vi "Measure Triggered Suply IV.vi"(0 "Supply Line Handle in":refnum<k15>, 1 "Channel Name":string, 11 "error in (no error)":errorcluster) -> (4 "Supply Line Handle out":refnum<k15>, 6 "Supply Line Measurements Results":T1, 15 "error out":errorcluster)   [LabVIEW 2016, in "SMU.lvlib"]
uses:
  SMU.lvlib
  <instrlib>/niDCPower/nidcpower.llb/niDCPower Send Software Edge Trigger - Signal.ctl
  Typedefs/IV Results.ctl
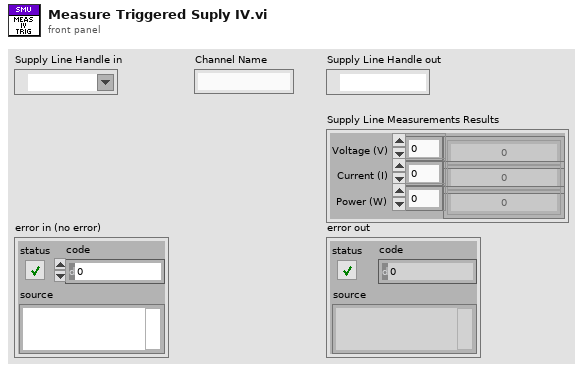
[diagram p1: front panel]
types:
  T1 = typedef "SMU.lvlib/IV Results.ctl" = cluster{"Voltage (V)":dbl[], "Current (I)":dbl[], "Power (W)":dbl[]}
  T2 = typedef "niDCPower Send Software Edge Trigger - Signal.ctl" = i32
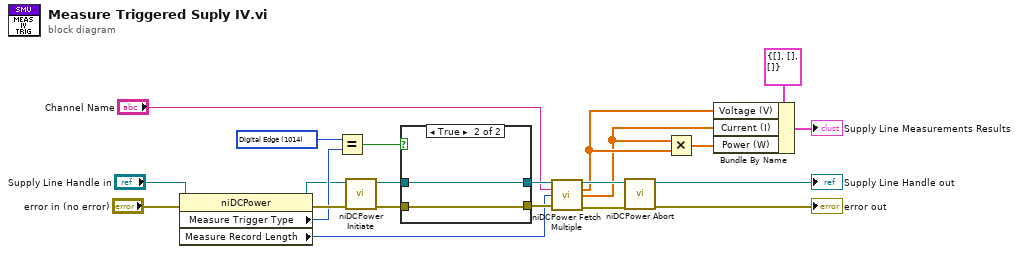
[diagram p0: block diagram]
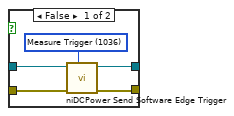
[diagram p2: hidden frame]
diagram:
  w13 = 1014 items=["Digital Edge"=1014, "Software Edge"=1015, "None"=1012] ("Triggers:Measure Trigger:Trigger Type")
  n1 = property class="niDCPower"(reference="Supply Line Handle in", error in="error in (no error)") -> (reference out=w3:refnum<k15>, error out=w18:errorcluster, "Measure Trigger Type"=w12:i32, "Measure Record Length"=w1:i32)
  n2 = Equal?(x=w13, y=w12) -> (x = y?=w14:bool)
  n3 = call <instrlib>:"niDCPower Initiate.vi"("error in (no error)"=w18, "instrument handle"=w3) -> ("error out"=w17:errorcluster, "instrument handle out"=w20:refnum<k15>)  [unwired: 8 in]
  n4 = case shown="True" w14 {
    tunnel: w20 -> [w26 w29]
    tunnel: [w25 w29] -> w19
    tunnel: [w24 w28] -> w16
    tunnel: w17 -> [w23 w28]
    frame False {
      w27 = T2 1036 items=["Start Trigger"=1034, "Source Trigger"=1035, "Measure Trigger"=1036, "Sequence Advance Trigger"=1037, "Pulse Trigger"=1053] ("signal")
      n5 = call <instrlib>:"niDCPower Send Software Edge Trigger.vi"("error in (no error)"=w23, "signal"=w27, "instrument handle"=w26) -> ("error out"=w24:errorcluster, "instrument handle out"=w25:refnum<k15>)  [unwired: 7 in]
    }
    frame True {
    }
  }
  n6 = call <instrlib>:"niDCPower Fetch Multiple.vi"("instrument handle"=w19, "channel name"="Channel Name", "count (1)"=w1, "error in (no error)"=w16) -> ("instrument handle out"=w21:refnum<k15>, "voltage measurements"=w11:dbl[], "current measurements"=w10:dbl[], "error out"=w15:errorcluster)  [unwired: 1 in, 7 out]
  n7 = call <instrlib>:"niDCPower Abort.vi"("error in (no error)"=w15, "instrument handle"=w21) -> ("error out"=→"error out":errorcluster, "instrument handle out"=→"Supply Line Handle out":refnum<k15>)  [unwired: 8 in]
  n8 = Multiply(x=w10, y=w11) -> (x*y=w5:dbl[])
  n9 = Bundle By Name(cluster=T1 {"Voltage (V)"=[], "Current (I)"=[], "Power (W)"=[]} ("Supply Line Measurements Results"), "Voltage (V)"=w11, "Current (I)"=w10, "Power (W)"=w5) -> (→"Supply Line Measurements Results":T1)
